vi "DAQ FGV.vi"(7 "Enum":T2, 8 "error in (no error)":errorcluster, 11 "Cluster":T1) -> (0 "error out":errorcluster, 3 "Cluster Out":T1)   [LabVIEW 2020]
uses:
  controls/DAQ FGV.ctl
  DAQLoop_Typedef.ctl
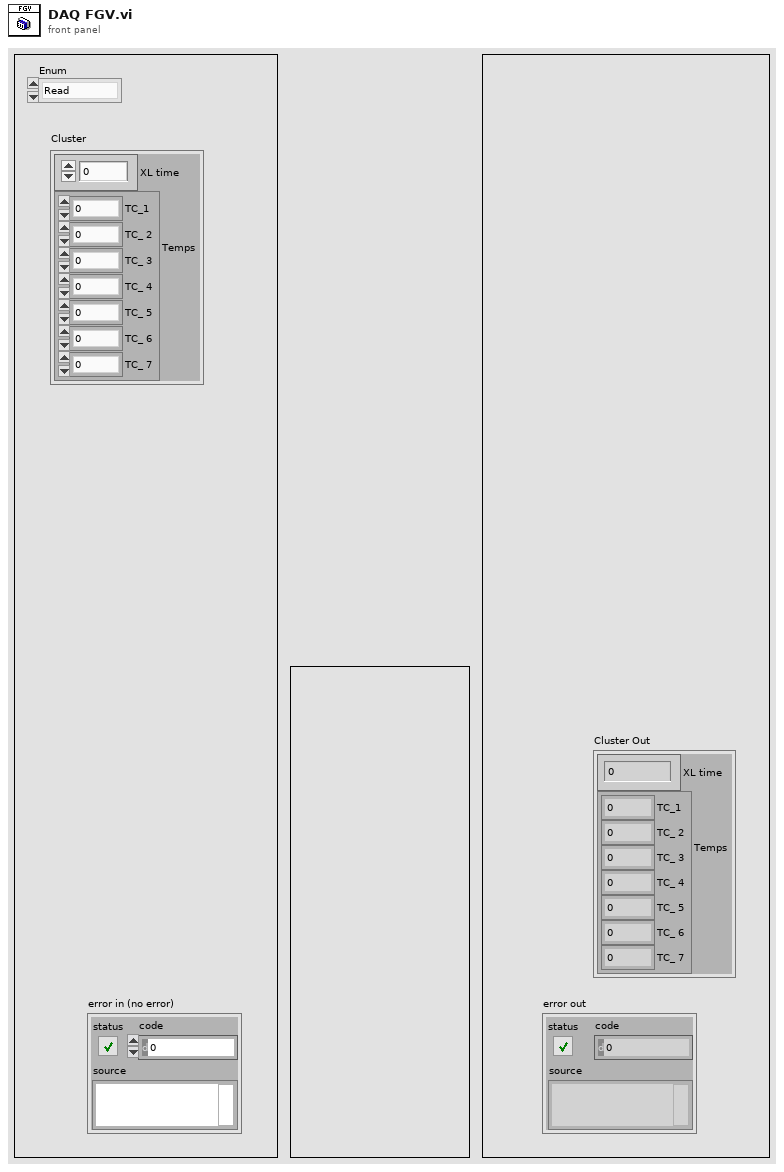
[diagram p1: front panel]
types:
  T1 = typedef "DAQLoop_Typedef.ctl" = cluster{"XL time":dbl, "Temps":cluster{"TC_1":dbl, "TC_ 2":dbl, "TC_ 3":dbl, "TC_ 4":dbl, "TC_ 5":dbl, "TC_ 6":dbl, "TC_ 7":dbl}}
  T2 = typedef "DAQ FGV.ctl" = enum16{"Read", "Pass"}
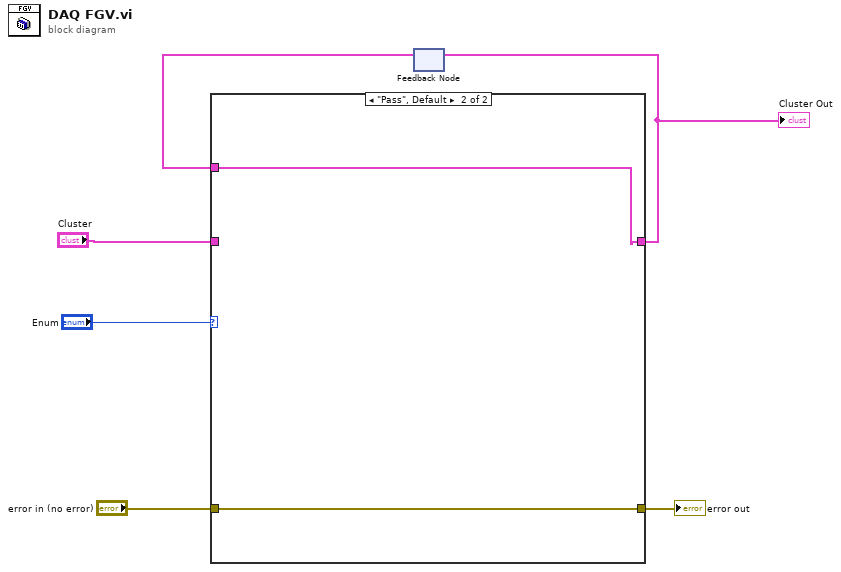
[diagram p0: block diagram]
diagram:
  n1 = feedback #1() -> (w2:T1)  [unwired: 1 in]
  n2 = case shown="\"Pass\", Default" "Enum" {
    tunnel: "error in (no error)" -> [w7 w10]
    tunnel: [w7 w10] -> w5
    tunnel: "Cluster" -> [w8 _]
    tunnel: [w8 w9] -> w3
    tunnel: w2 -> [_ w9]
    frame "Read" {
    }
    frame "Pass", Default {
    }
  }
  "error out" <- w5
  "Cluster Out" <- w3
  n3 = feedback-in #1(w3) -> ()
